vi "Tree Control Example.vi"   [LabVIEW 2025]
uses:
  <vilib>/Utility/EditLVProj/Edit LVProj.lvlib
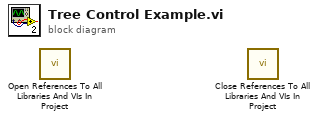
[diagram p0: block diagram]
diagram:
  n1 = call <vilib>:"Open References To All Libraries And VIs In Project.vi"() -> ()  [unwired: 9 in, 3 out]
  n2 = call <vilib>:"Close References To All Libraries And VIs In Project.vi"() -> ()  [unwired: 11 in, 1 out]
